vi "Benchmark_Streaming_uBroker.vi"() -> ()   [LabVIEW 2021]
uses:
  Bin/uFramework.lvlibp/uBroker/uBroker.lvclass
  _TestClasses/Test_uActor_StreamingSubscriber/Test_uActor_StreamingSubscriber.lvclass
  360130bd-e545-437f-86ab-c1c949312b85.vi
  6f74bf88-0135-4991-9169-aef5c84be21e.vi
  81a9c915-3656-48b0-9691-fbfefa660d7c.vi
  Bin/uFramework.lvlibp/uTransport_Event/uTransport_Event.lvclass
  U:/Projects/uFramework/Bin/uFramework.lvlibp/uTransport/uTransport.lvclass
  Bin/uFramework.lvlibp/uTransport_Queue/uTransport_Queue.lvclass
  Bin/uFramework.lvlibp/uTransport_uActor/uTransport_uActor.lvclass
  Bin/uFramework.lvlibp/uPolicy/Write uNotifyMode.vi
  Bin/uData.lvlibp/Set Tag.vi
  Bin/uData.lvlibp/Get Tag.vi
  Bin/uData.lvlibp/uData.lvclass
  Bin/uFramework.lvlibp/uActor/uActor.lvclass
  Bin/uFramework.lvlibp/uClient_Publisher/uClient_Publisher.lvclass
  U:/Projects/uFramework/Bin/uFramework.lvlibp/uTransport_Event/uTransport_Event.lvclass
  Bin/uFramework.lvlibp/uMsg/uMsg.lvclass
  Bin/uFramework.lvlibp/uClient_Subscriber/uClient_Subscriber.lvclass
  U:/Projects/uFramework/Bin/uFramework.lvlibp/uActor/uActor.lvclass
  U:/Projects/uFramework/Bin/uFramework.lvlibp/uBroker/uBroker.lvclass
  U:/Projects/uFramework/Testers/_TestClasses/Test_uActor_StreamingSubscriber/Test_uActor_StreamingSubscriber.lvclass
  U:/Projects/uFramework/Bin/uFramework.lvlibp/uTransport_uActor/uTransport_uActor.lvclass
  U:/Projects/uFramework/Bin/uFramework.lvlibp/uTransport_Queue/uTransport_Queue.lvclass
panel:
  out "i (E)":i32
  out "i (Q)":i32
  out "Latency (ms) E":u32
  out "Latency (ms) Q":u32
  out "Received (E)":i32
  out "Received (Q)":i32
  out "Sent":i32
  in  "Rate":i32
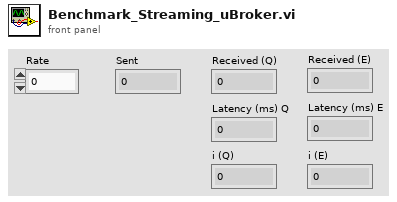
[diagram p1: front panel]
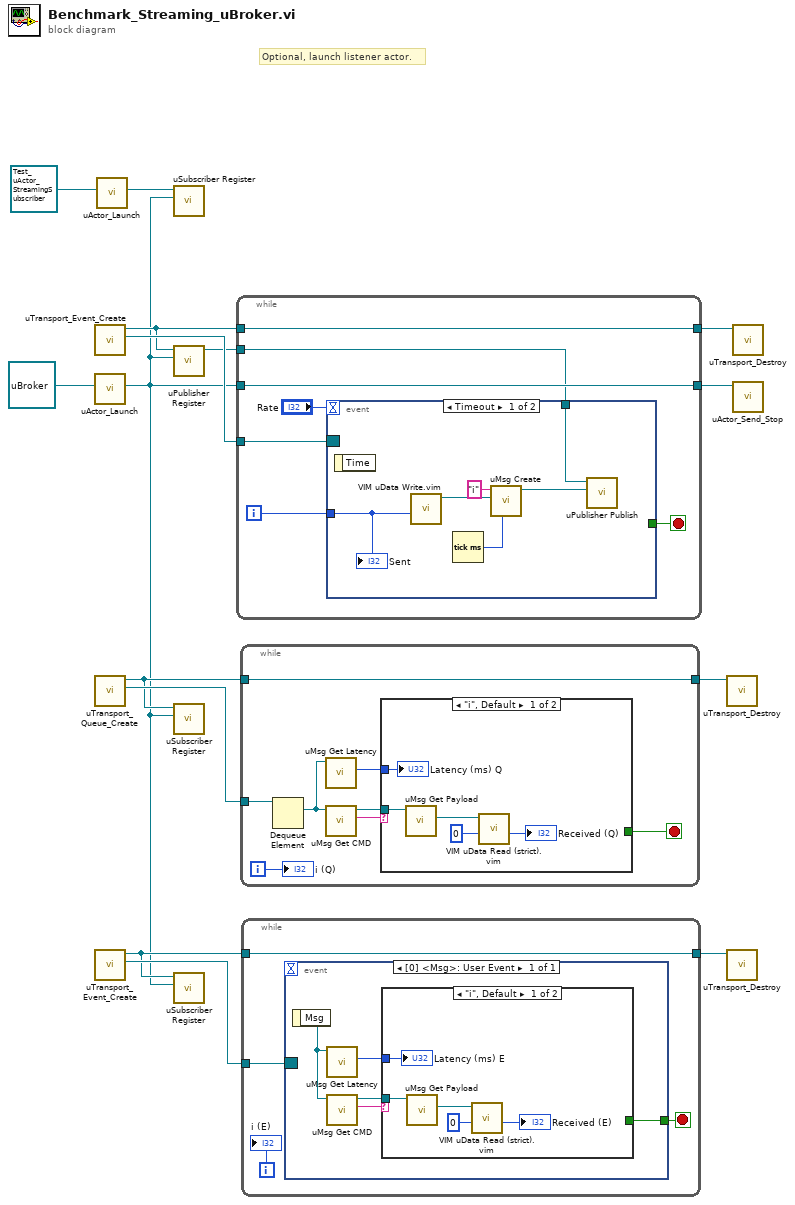
[diagram p0: block diagram]
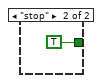
[diagram p2: hidden frame]
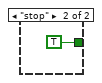
[diagram p3: hidden frame]
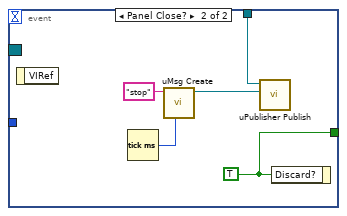
[diagram p4: hidden frame]
diagram:
  # "Optional, launch listener actor."
  n1 = call "uTransport_Event_Create.vi"() -> ("Event:uMsg"=w13:refnum<event-registration>, "uTransport_Event out"=w11:refnum<class "uTransport_Event.lvclass">)  [unwired: 9 in, 1 out]
  n2 = call "uActor_Launch.vi"("Actor to Launch"=refnum<class "uBroker.lvclass"> refnum) -> ("uTransport_uActor"=w3:refnum<class "uTransport_uActor.lvclass">)  [unwired: 8 in, 2 out]
  n3 = call "uTransport_Queue_Create.vi"() -> ("queue"=w8:refnum<queue>, "uTransport_Queue out"=w5:refnum<class "uTransport_Queue.lvclass">)  [unwired: 9 in, 1 out]
  n4 = call "uTransport_Event_Create.vi"() -> ("Event:uMsg"=w6:refnum<event-registration>, "uTransport_Event out"=w4:refnum<class "uTransport_Event.lvclass">)  [unwired: 9 in, 1 out]
  n5 = call "uActor_Launch.vi"("Actor to Launch"=refnum<class "Test_uActor_StreamingSubscriber.lvclass"> refnum ("Test_uActor_StreamingSubscriber.lvclass")) -> ("uTransport_uActor"=w2:refnum<class "uTransport_uActor.lvclass">)  [unwired: 8 in, 2 out]
  n6 = call "uSubscriber Register.vi"("Broker"=w3, "Subscriber's uTransport"=w2) -> ()  [unwired: 9 in, 1 out]
  n7 = call "uPublisher Register.vi"("Broker"=w3, "Publisher's uTransport"=w11) -> ("uClient_Publisher out"=w10:refnum<class "uClient_Publisher.lvclass">)  [unwired: 8 in, 1 out]
  n8 = call "uSubscriber Register.vi"("Broker"=w3, "Subscriber's uTransport"=w5) -> ()  [unwired: 9 in, 1 out]
  n9 = call "uSubscriber Register.vi"("Broker"=w3, "Subscriber's uTransport"=w4) -> ()  [unwired: 9 in, 1 out]
  n10 = while {
    tunnel: [w20] -> w14
    tunnel: w3 -> [w20]
    tunnel: w13 -> [w19]
    tunnel: w11 -> [w18]
    tunnel: [w18] -> w12
    tunnel: w10 -> [w17]
    i -> [w16]
    stop <- w22 stop-if-true
    n11 = event shown="[0] Timeout" {
      selector: w19 -> [_ _]
      dyn-events: _ -> [_ _]
      timeout: "Rate" -> [_ _]
      tunnel: [_ w33] -> w22
      tunnel: w17 -> [w28 w30]
      tunnel: w16 -> [w26 _]
      event Timeout {
        n12 = event-data() -> ()  [unwired: 1 in, 1 out]
        n13 = call "VIM uData Write.vim"("value"=w26) -> ("uData out"=w27:refnum<class "uData.lvclass">)  [unwired: 8 in, 2 out]
        n14 = Tick Count (ms)() -> (millisecond timer value=w23:u32)
        n15 = call "uMsg Create.vi"("Timestamp (NULL)"=w23, "Payload"=w27, "CMD"="i") -> ("uMsg out"=w24:refnum<class "uMsg.lvclass">)  [unwired: 7 in, 1 out]
        n16 = call "uPublisher Publish.vi"("uMsg"=w24, "uClient_Publisher in"=w28) -> ()  [unwired: 8 in, 2 out]
        "Sent" <- w26
      }
      event Panel Close? {
        w33 = TRUE ("Discard?")
        n17 = event-data() -> ()  [unwired: 1 in, 1 out]
        n18 = Tick Count (ms)() -> (millisecond timer value=w29:u32)
        n19 = call "uMsg Create.vi"("Timestamp (NULL)"=w29, "CMD"="stop") -> ("uMsg out"=w32:refnum<class "uMsg.lvclass">)  [unwired: 8 in, 1 out]
        n20 = call "uPublisher Publish.vi"("uMsg"=w32, "uClient_Publisher in"=w30) -> ()  [unwired: 8 in, 2 out]
        n21 = event-data("Discard?"=w33) -> ()  [unwired: 1 in, 1 out]
      }
    }
  }
  n22 = while {
    tunnel: w5 -> [w41]
    tunnel: [w41] -> w9
    tunnel: w8 -> [w40]
    i -> [w34]
    stop <- w38 stop-if-true
    n23 = Dequeue Element(queue=w40) -> (element=w36:refnum<class "uMsg.lvclass">)  [unwired: 2 in, 3 out]
    n24 = call "uMsg Get Latency.vi"("uMsg in"=w36) -> ("Latency (ms)"=w35:u32)  [unwired: 8 in, 2 out]
    n25 = call "uMsg Get CMD.vi"("uMsg in"=w36) -> ("CMD"=w39:string, "uMsg out"=w37:refnum<class "uMsg.lvclass">)  [unwired: 8 in, 1 out]
    n26 = case shown="\"i\", Default" w39 {
      tunnel: [_ TRUE] -> w38
      tunnel: w37 -> [w46 _]
      tunnel: w35 -> [w44 _]
      frame "i", Default {
        n27 = call "uMsg Get Payload.vi"("uMsg in"=w46) -> ("uData"=w45:refnum<class "uData.lvclass">)  [unwired: 8 in, 2 out]
        n28 = call "VIM uData Read (strict).vim"("default value"=0, "uData in"=w45) -> ("value"=→"Received (Q)":i32)  [unwired: 6 in, 3 out]
        "Latency (ms) Q" <- w44
      }
      frame "stop" {
      }
    }
    "i (Q)" <- w34
  }
  n29 = while {
    tunnel: w4 -> [w51]
    tunnel: [w51] -> w7
    tunnel: w6 -> [w49]
    i -> [w48]
    stop <- w50 stop-if-true
    n30 = event shown="[0] <Msg>: User Event" {
      selector: w49 -> [_]
      dyn-events: _ -> [_]
      timeout: _ -> [_]
      tunnel: [w55] -> w50
      event User Event {
        n31 = event-data() -> ("Msg"=w52:refnum<class "uMsg.lvclass">)  [unwired: 1 in]
        n32 = call "uMsg Get Latency.vi"("uMsg in"=w52) -> ("Latency (ms)"=w53:u32)  [unwired: 8 in, 2 out]
        n33 = call "uMsg Get CMD.vi"("uMsg in"=w52) -> ("CMD"=w56:string, "uMsg out"=w54:refnum<class "uMsg.lvclass">)  [unwired: 8 in, 1 out]
        n34 = case shown="\"i\", Default" w56 {
          tunnel: [_ TRUE] -> w55
          tunnel: w54 -> [w61 _]
          tunnel: w53 -> [w58 _]
          frame "i", Default {
            n35 = call "uMsg Get Payload.vi"("uMsg in"=w61) -> ("uData"=w60:refnum<class "uData.lvclass">)  [unwired: 8 in, 2 out]
            n36 = call "VIM uData Read (strict).vim"("default value"=0, "uData in"=w60) -> ("value"=→"Received (E)":i32)  [unwired: 6 in, 3 out]
            "Latency (ms) E" <- w58
          }
          frame "stop" {
          }
        }
      }
    }
    "i (E)" <- w48
  }
  n37 = call-dynamic "uTransport_Destroy.vi"("uTransport_Queue in"=w9) -> ()  [unwired: 10 in, 1 out]
  n38 = call-dynamic "uTransport_Destroy.vi"("uTransport_Event in"=w7) -> ()  [unwired: 10 in, 1 out]
  n39 = call-dynamic "uTransport_Destroy.vi"("uTransport_Event in"=w12) -> ()  [unwired: 10 in, 1 out]
  n40 = call "uActor_Send_Stop.vi"("uActor Transport"=w14) -> ()  [unwired: 10 in, 1 out]
